vi "ChrolisExample.vi"() -> ()   [LabVIEW 2023]
panel:
  out "Color LED 5":string
  out "Color LED 3":string
  out "Color LED 2":string
  out "Color LED 1":string
  out "Color LED 4":string
  out "Color LED 6":string
  in  "Stopp":bool
  in  "Enable LED 6":bool
  in  "Enable LED 4":bool
  in  "Enable LED 2":bool
  in  "Enable LED 1":bool
  in  "Enable LED 3":bool
  in  "Enable LED 5":bool
  in  "Brightness LED 6":i16(slide) caption="Brightness LED 6 (0)" scale=0.0..1000.0
  in  "Brightness LED 2":i16(slide) caption="Brightness LED 2 (0)" scale=0.0..1000.0
  in  "Brightness LED 4":i16(slide) caption="Brightness LED 4 (0)" scale=0.0..1000.0
  in  "Brightness LED 1":i16(slide) caption="Brightness LED 1 (0)" scale=0.0..1000.0
  in  "Brightness LED 3":i16(slide) caption="Brightness LED 3 (0)" scale=0.0..1000.0
  in  "Brightness LED 5":i16(slide) caption="Brightness LED 5 (0)" scale=0.0..1000.0
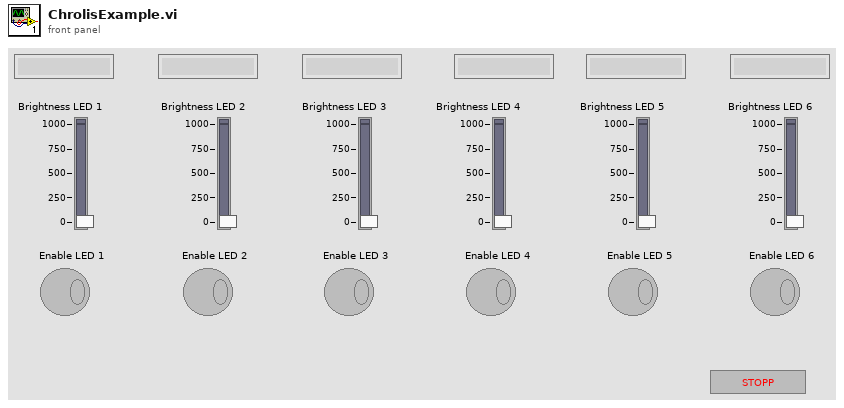
[diagram p1: front panel]
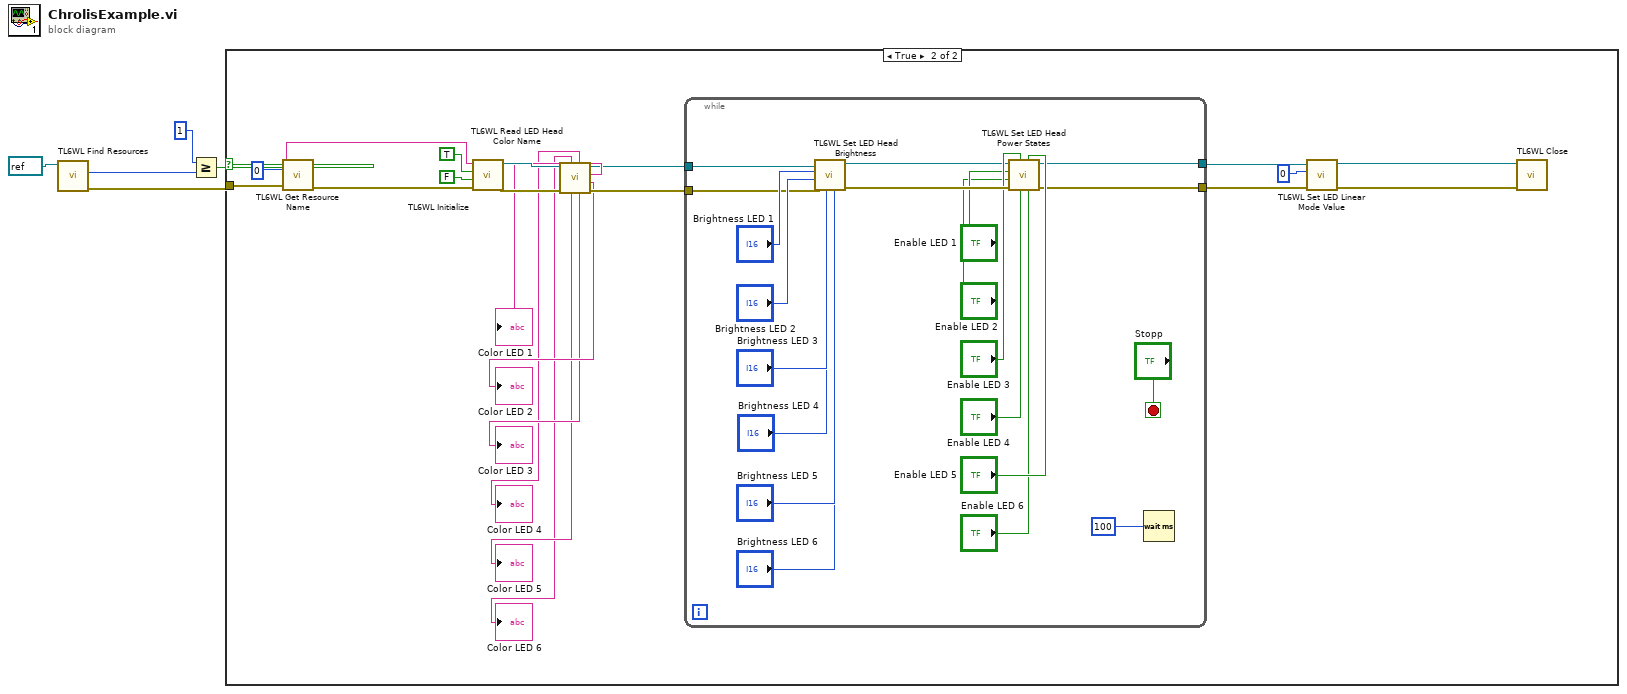
[diagram p0: block diagram]
diagram:
  n1 = call "TL6WL Find Resources.vi"("instrument handle"=refnum<visa-resource-name> refnum) -> ("error out"=w1:errorcluster, "Device Count"=w4:u32)  [unwired: 8 in, 1 out]
  n2 = Greater Or Equal?(x=u32 1 ("y"), y=w4) -> (x >= y?=w2:bool)
  n3 = case shown="True" w2 {
    tunnel: w1 -> [_ w26]
    frame False {
    }
    frame True {
      n4 = call "TL6WL Get Resource Name.vi"("error in (no error)"=w26, "Device Index"=u32 0) -> ("error out"=w24:errorcluster, "Resource Name"=w23:string)  [unwired: 7 in, 1 out]
      n5 = call "TL6WL Initialize.vi"("error in (no error)"=w24, "Reset Device (Reset Device)"=FALSE, "ID Query (Do Query)"=TRUE, "resource name"=w23) -> ("error out"=w15:errorcluster, "instrument handle out"=w14:refnum<visa-resource-name>)  [unwired: 6 in]
      n6 = call "TL6WL Read LED Head Color Name.vi"("error in (no error)"=w15, "instrument handle"=w14) -> ("error out"=w13:errorcluster, "Color LED 2"=→"Color LED 2":string, "Color LED 1"=→"Color LED 1":string, "instrument handle out"=w10:refnum<visa-resource-name>, "Color LED 3"=→"Color LED 3":string, "Color LED 4"=→"Color LED 4":string, "Color LED 5"=→"Color LED 5":string, "Color LED 6"=→"Color LED 6":string)  [unwired: 2 in]
      n7 = while {
        tunnel: [w31] -> w20
        tunnel: [w30] -> w19
        tunnel: w13 -> [w28]
        tunnel: w10 -> [w27]
        stop <- "Stopp" stop-if-true
        n8 = call "TL6WL Set LED Head Brightness.vi"("Brightness LED 6 (0)"="Brightness LED 6", "Brightness LED 5 (0)"="Brightness LED 5", "Brightness LED 4 (0)"="Brightness LED 4", "Brightness LED 3 (0)"="Brightness LED 3", "error in (no error)"=w28, "Brightness LED 2 (0)"="Brightness LED 2", "Brightness LED 1 (0)"="Brightness LED 1", "instrument handle"=w27) -> ("error out"=w40:errorcluster, "instrument handle out"=w33:refnum<visa-resource-name>)  [unwired: 2 in]
        n9 = call "TL6WL Set LED Head Power States.vi"("Enable LED 6"="Enable LED 6", "Enable LED 5"="Enable LED 5", "Enable LED 4"="Enable LED 4", "Enable LED 3"="Enable LED 3", "error in (no error)"=w40, "Enable LED 2"="Enable LED 2", "Enable LED 1"="Enable LED 1", "instrument handle"=w33) -> ("error out"=w30:errorcluster, "instrument handle out"=w31:refnum<visa-resource-name>)  [unwired: 2 in]
        n10 = Wait (ms)(milliseconds to wait=u32 100 ("Zu wartende ms")) -> ()  [unwired: 1 out]
      }
      n11 = call "TL6WL Set LED Linear Mode Value.vi"("error in (no error)"=w19, "Brightness (0)"=u16 0, "instrument handle"=w20) -> ("error out"=w16:errorcluster, "instrument handle out"=w17:refnum<visa-resource-name>)  [unwired: 7 in]
      n12 = call "TL6WL Close.vi"("error in (no error)"=w16, "instrument handle"=w17) -> ()  [unwired: 9 in, 1 out]
    }
  }
